vi "all-signals-expressvi-to-TDMS-01-inloop.vi"() -> ()   [LabVIEW 2018]
panel:
  in  "Dateiname":string="test.tdms"
  in  "Dateipfad":path=path "C:/Users/lauri/OneDrive/Dokumente/Uni/HTW/Diplomarbeit/Versuchsstand neu/labview/messungen"
  in  "Stop Measurement (F)":bool caption="Messung stoppen, Counter schreiben (F)"
  in  "Clear Charts":bool
  in  "Messzeit in ms":u32=100 min=10 max=1000 step=10
  out "Bremsmoment":waveform(dbl)(graph)
  out "Strom, Spannung, elektrische Leistung":dynamicdata(graph)
  out "Counter/Messzeit":waveform(dbl)(graph)
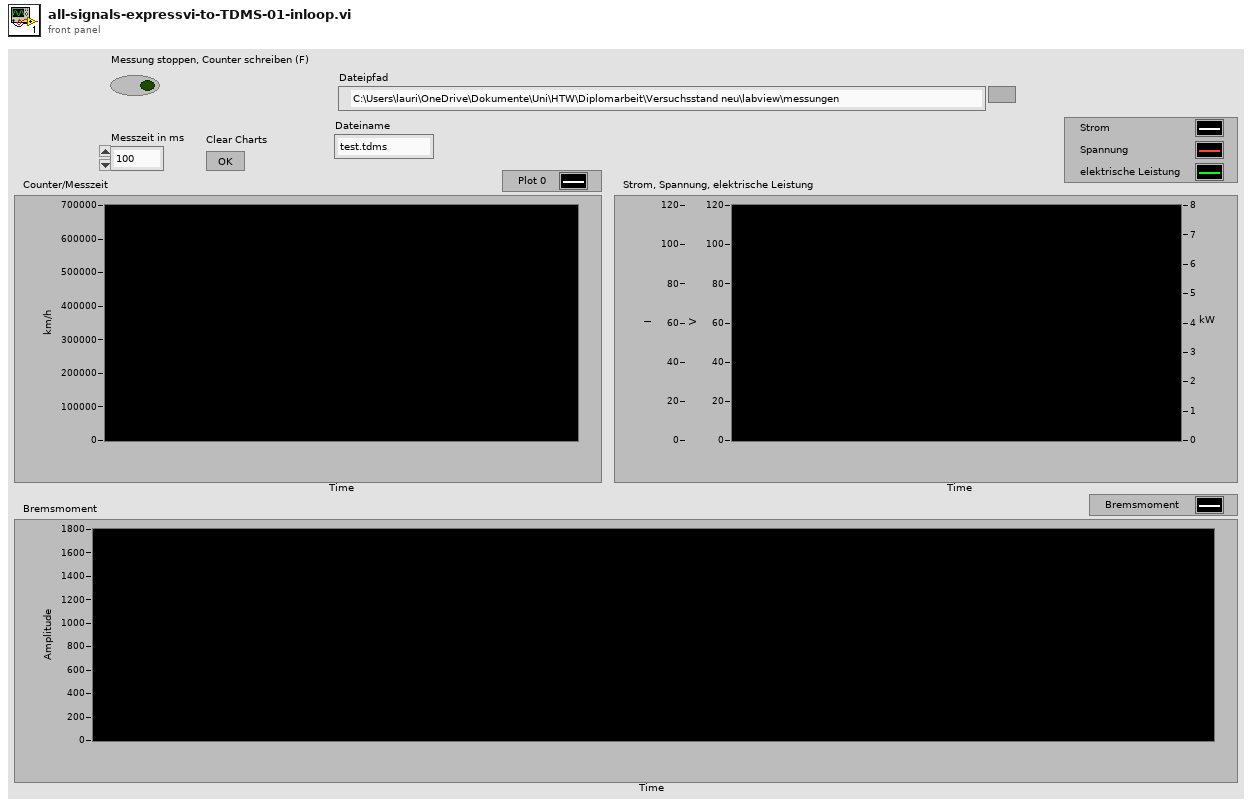
[diagram p1: front panel]
types:
  T1 = enum16{"open", "open or create", "create or replace", "create", "open (read-only)"}
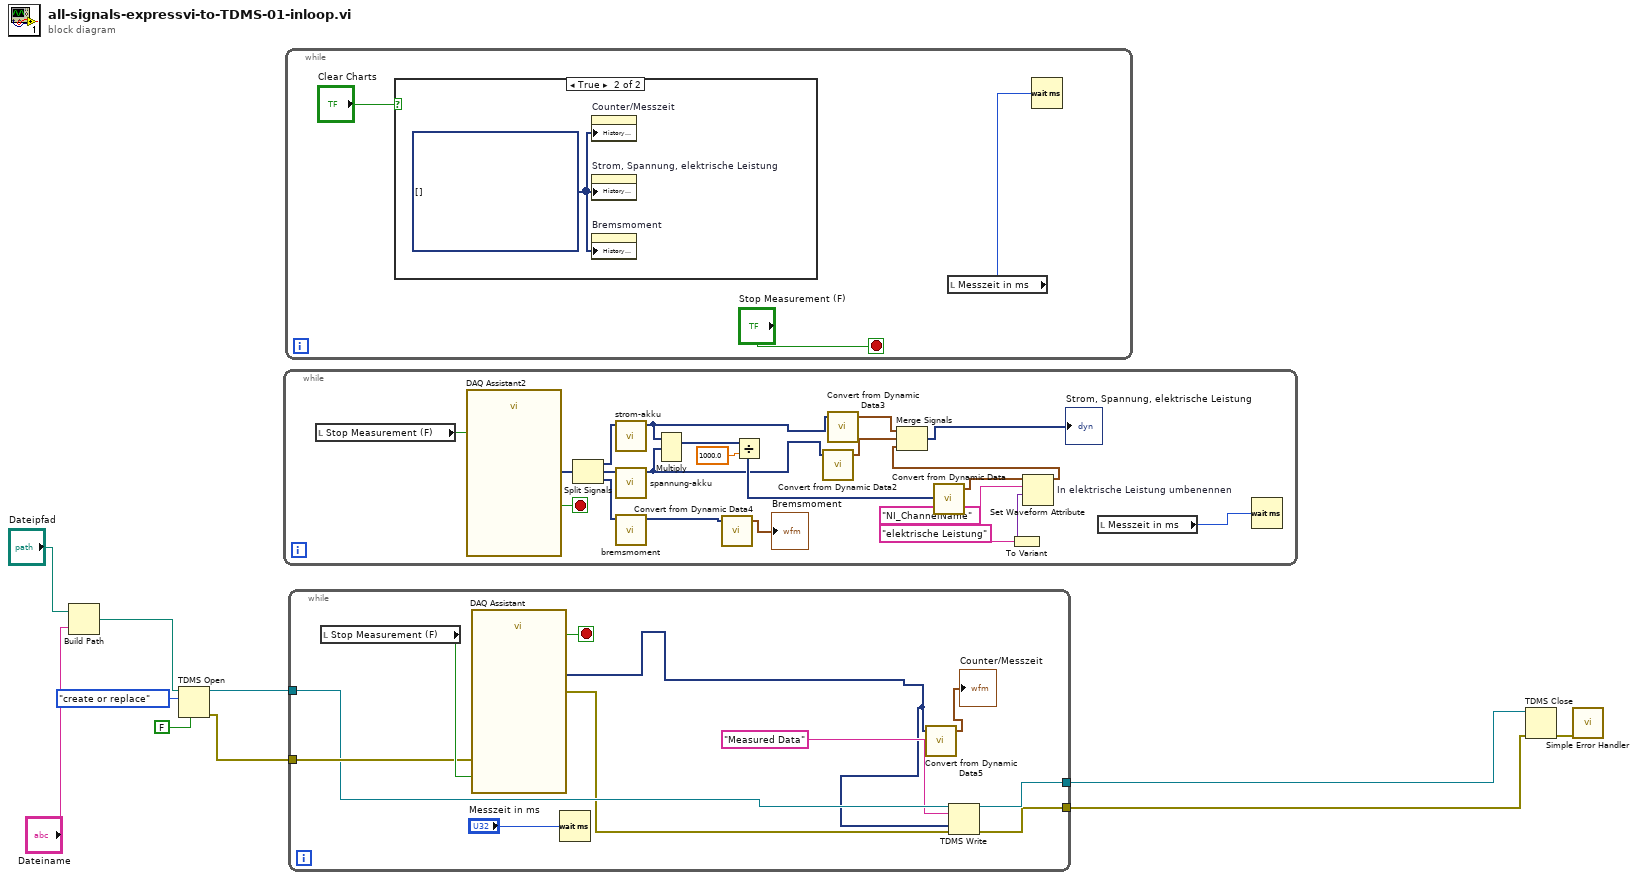
[diagram p0: block diagram]
diagram:
  n1 = Build Path(base path="Dateipfad", name or relative path="Dateiname") -> (appended path=w7:path)
  n2 = TDMS Open(6:FALSE ("disable buffering? (T)"), 10:T1."create or replace" ("operation (0:open)"), 11:w7) -> (0:w10:errorcluster, 3:w3:refnum<k34>)  [unwired: 4 in]
  n3 = while {
    stop <- w28 stop-if-true
    n4 = local read "Stop Measurement (F)"() -> (w25:bool)
    n5 = call "DAQ Assistant2"("stop (F)"=w25) -> ("data"=w29:dynamicdata, "stopped"=w28:bool)  [unwired: 15 in, 2 out]
    n6 = Split Signals(w29) -> (w32:dynamicdata, w31:dynamicdata, w30:dynamicdata)  [unwired: 3 in]
    n7 = call "strom-akku.vi"("Dynamic Data"=w32) -> ("Filtered Signal"=w16:dynamicdata)  [unwired: 10 in]
    n8 = call "spannung-akku.vi"("Dynamic Data in"=w31) -> ("Dynamic Data out"=w18:dynamicdata)  [unwired: 10 in]
    n9 = call "bremsmoment.vi"("Dynamic Data in"=w30) -> ("Dynamic Data out"=w14:dynamicdata)  [unwired: 10 in]
    n10 = Multiply(1:w18, 2:w16) -> (0:w26:dynamicdata)  [unwired: 1 in, 1 out]
    n11 = call "Convert from Dynamic Data4"("Dynamic Data Type"=w14) -> ("Waveform"=→"Bremsmoment":waveform(dbl))  [unwired: 3 in]
    n12 = Divide(x=w26, y=1000.0) -> (x/y=w24:dynamicdata)
    n13 = call "Convert from Dynamic Data2"("Dynamic Data Type"=w18) -> ("Waveform"=w17:waveform(dbl))  [unwired: 3 in]
    n14 = call "Convert from Dynamic Data3"("Dynamic Data Type"=w16) -> ("Waveform"=w15:waveform(dbl))  [unwired: 3 in]
    n15 = call "Convert from Dynamic Data"("Dynamic Data Type"=w24) -> ("Waveform"=w20:waveform(dbl))  [unwired: 3 in]
    n16 = To Variant(anything="elektrische Leistung") -> (Variant=w23:variant)
    n17 = Set Waveform Attribute "In elektrische Leistung umbenennen"(5:w23, 6:"NI_ChannelName" ("name"), 7:w20) -> (3:w19:waveform(dbl))  [unwired: 1 in, 2 out]
    n18 = Merge Signals "Merge Signals"(w15, w17, w19) -> (→"Strom, Spannung, elektrische Leistung":dynamicdata)
    n19 = local read "Messzeit in ms"() -> (w11:u32)
    n20 = Wait (ms)(milliseconds to wait=w11) -> ()  [unwired: 1 out]
  }
  n21 = while {
    stop <- "Stop Measurement (F)" stop-if-true
    n22 = case shown="True" "Clear Charts" {
      frame False {
      }
      frame True {
        w36 = dynamicdata[] [] ("History Data")
        n23 = property on="Counter/Messzeit" class="WFChart (strict)"("History Data"=w36) -> ()  [unwired: 2 in, 2 out]
        n24 = property on="Strom, Spannung, elektrische Leistung" class="WFChart (strict)"("History Data"=w36) -> ()  [unwired: 2 in, 2 out]
        n25 = property on="Bremsmoment" class="WFChart (strict)"("History Data"=w36) -> ()  [unwired: 2 in, 2 out]
      }
    }
    n26 = local read "Messzeit in ms"() -> (w33:u32)
    n27 = Wait (ms)(milliseconds to wait=w33) -> ()  [unwired: 1 out]
  }
  n28 = while {
    tunnel: w10 -> [w45]
    tunnel: w3 -> [w43]
    tunnel: [w40] -> w2
    tunnel: [w39] -> w1
    stop <- w47 stop-if-true
    n29 = local read "Stop Measurement (F)"() -> (w46:bool)
    n30 = call "DAQ Assistant"("error in"=w45, "stop (F)"=w46) -> ("data"=w37:dynamicdata, "stopped"=w47:bool, "error out"=w41:errorcluster)  [unwired: 14 in, 1 out]
    n31 = Wait (ms)(milliseconds to wait="Messzeit in ms") -> ()  [unwired: 1 out]
    n32 = call "Convert from Dynamic Data5"("Dynamic Data Type"=w37) -> ("Waveform"=→"Counter/Messzeit":waveform(dbl))  [unwired: 3 in]
    n33 = TDMS Write(0:w43, 5:"Measured Data" ("group name in (Untitled)"), 9:w37, 11:w41) -> (4:w40:refnum<k34>, 15:w39:errorcluster)  [unwired: 2 in, 2 out]
  }
  n34 = TDMS Close(8:w1, 11:w2) -> (0:w4:errorcluster)  [unwired: 1 out]
  n35 = call <vilib>:"Simple Error Handler.vi"("error in (no error)"=w4) -> ()  [unwired: 2 in, 7 out]
